vi "Stop Core.vi"(10 "final error code":i32, 11 "Nested in":refnum<class "Model_AMC.lvclass">) -> (3 "Nested out":refnum<class "Model_AMC.lvclass">)   [LabVIEW 2021, in "Model_AMC.lvclass"]
doc: "(<B>Filename</B>: Actor Framework.lvlib:Actor.lvclass:Stop Core.vi)\n\nDefines what the actor does before it stops. Use the <B>final error code</B> input to determine whether the actor shut down in response to an error.\n\nBy default, this method does nothing. A descendant class may override it to define behavior, such as shutting down any processes the actor initiated in its override of the Actor Core method."
uses:
  Model_AMC.lvclass
  Model_AMC.lvclass/Model_AMC.ctl
  <userlib>/John_Lib/AbstractActorTemplate/AbstractActorTemplate/UIActorTop.lvclass
  aa7f3e9f-24d5-48c5-94fc-7e7a2b89817f.vi
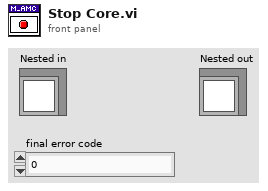
[diagram p1: front panel]
types:
  T1 = typedef "AMC_FW.lvlib/Queue.ctl" = cluster{"Q":T2, "Name":string}
  T2 = typedef "AMC_FW.lvlib/Message Queue.ctl" = refnum<queue>
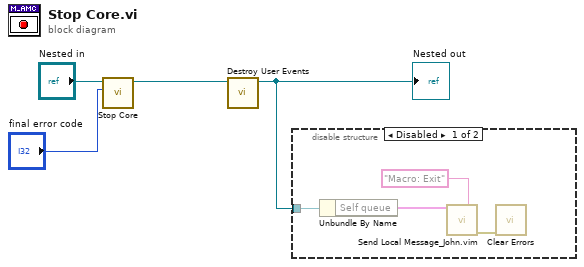
[diagram p0: block diagram]
diagram:
  n1 = call-parent "Stop Core.vi"("final error code"="final error code", "Nested in"="Nested in") -> ("Nested out"=w2:refnum<class "Model_AMC.lvclass">)  [unwired: 9 in]
  n2 = call "Destroy User Events.vi"("UI Template in"=w2) -> ("UI Template out"=w1:refnum<class "Model_AMC.lvclass">)  [unwired: 10 in]
  "Nested out" <- w1
  n3 = disable-structure shown="Disabled" {
    disable-tunnel: w1 -> [w5 _]
    frame Disabled {
      n4 = Unbundle By Name(w5) -> ("Self queue"=w8:T1)
      n5 = call "Send Local Message_John.vim"("Queue In"=w8, "Elements in Front"="Macro: Exit") -> ("error out"=w7:errorcluster)  [unwired: 11 in, 2 out]
      n6 = call <vilib>:"Clear Errors.vi"("error in (no error)"=w7) -> ()  [unwired: 5 in, 2 out]
    }
    frame Enabled {
    }
  }
